vi "Save Config.vi"(8 "error in (no error)":errorcluster, 11 "Server Creator Data":T1) -> (0 "error out":errorcluster)   [LabVIEW 2025, in "Tools.lvlib"]
uses:
  Tools.lvlib
  Server Creator Data.ctl
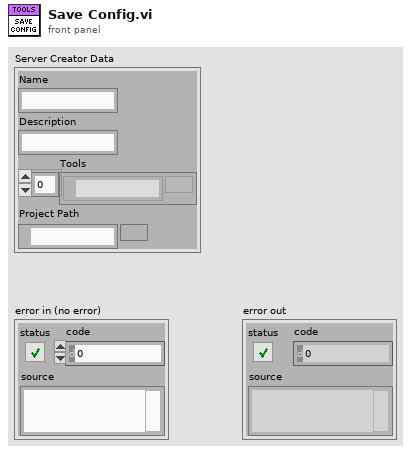
[diagram p1: front panel]
types:
  T1 = typedef "Tools.lvlib/Server Creator Data.ctl" = cluster{"Name":string, "Description":string, "Tools":path[], "Project Path":path}
  T2 = enum16{"open", "replace", "create", "open or create", "replace or create", "replace or create with confirmation"}
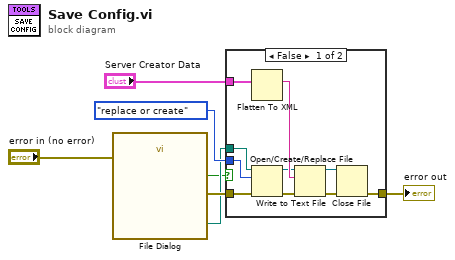
[diagram p0: block diagram]
diagram:
  n1 = call "File Dialog"("error in"="error in (no error)") -> ("selected path"=w2:path, "cancelled"=w1:bool, "error out"=w7:errorcluster)  [unwired: 11 in, 1 out]
  n2 = case shown="False" w1 {
    tunnel: w7 -> [w17 w18]
    tunnel: [w16 w18] -> w5
    tunnel: "Server Creator Data" -> [w14 _]
    tunnel: T2."replace or create" ("operation (0:open)") -> [w13 _]
    tunnel: w2 -> [w12 _]
    frame False {
      n3 = Flatten To XML(6:w14) -> (2:w15:string)
      n4 = Open/Create/Replace File(file path (use dialog)=w12, error in=w17, operation (0:open)=w13) -> (refnum out=w8:refnum<file>, error out=w9:errorcluster)  [unwired: 3 in, 1 out]
      n5 = Write to Text File(file (use dialog)=w8, text=w15, error in=w9) -> (refnum out=w10:refnum<file>, error out=w11:errorcluster)  [unwired: 1 in, 1 out]
      n6 = Close File(refnum=w10, error in=w11) -> (error out=w16:errorcluster)  [unwired: 1 out]
    }
    frame True {
    }
  }
  "error out" <- w5
